vi "Calculate Joint Vectors.vi"(8 "Error In":errorcluster, 9 "Body Index":i32, 10 "Joints":T2, 11 "KinectSensor References":T3) -> (0 "Error Out":errorcluster, 1 "Joint 2-3 Vector":dbl[](array[numeric]), 2 "Joint 1-2 Vector":dbl[](array[numeric]), 3 "KinectSensor References":T3, 4 "Angle Between Bones (deg)":dbl)   [LabVIEW 2011, in "KinectOne.lvlib"]
doc: "Given 3 joints calculate the vector from joint 1 to 2 and from joint 2 to 3 as well as the angel between the two 'bone' vectors in degrees."
uses:
  KinectOne.lvlib
  Private/Type Defs/KinectSensor References.ctl
  Microsoft.Kinect
  C:/github/makerhub/KinectOne/LabVIEW/vi.lib/MakerHub/KinectOne/Private/Libs/BodyFrameDataInterface.dll
  Private/Libs/BodyFrameDataInterface.dll
  Private/Type Defs/JointType.ctl
  <vilib>/Analysis/baseanly.llb/Unit Vector (DBL).vi
  <vilib>/Analysis/NI_AALBase.lvlib
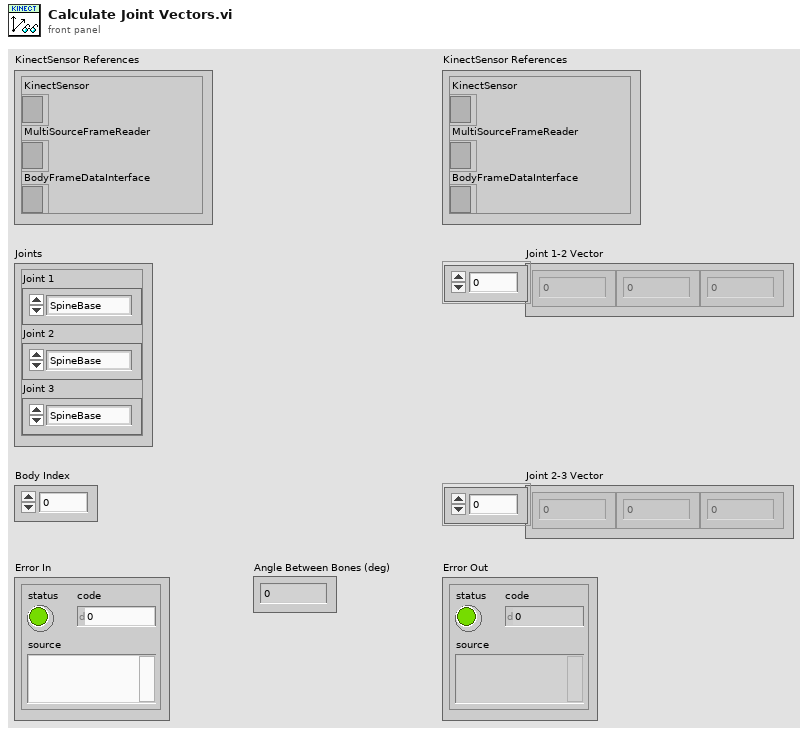
[diagram p1: front panel]
types:
  T1 = typedef "KinectOne.lvlib/JointType.ctl" = enum16{"SpineBase", "SpineMid", "Neck", "Head", "ShoulderLeft", "ElbowLeft", "WristLeft", "HandLeft", "ShoulderRight", "ElbowRight", "WristRight", "HandRight", "HipLeft", "KneeLeft", "AnkleLeft", "FootLeft", "HipRight", "KneeRight", "AnkleRight", "FootRight", "SpineShoulder", "HandTipLeft", "ThumbLeft", "HandTipRight", "ThumbRight"}
  T2 = cluster{"Joint 1":T1, "Joint 2":T1, "Joint 3":T1}
  T3 = typedef "KinectOne.lvlib/KinectSensor References.ctl" = cluster{"KinectSensor":refnum<k24>, "MultiSourceFrameReader":refnum<k24>, "BodyFrameDataInterface":refnum<k24>}
  T4 = typedef "KinectOne.lvlib/Joint Position.ctl" = cluster{"Camera Space":cluster{"X":dbl, "Y":dbl, "Z":dbl}, "Color Space":cluster{"X":dbl, "Y":dbl}, "Depth Space":cluster{"X":dbl, "Y":dbl}, "Tracking State":enum16{"NotTracked", "Inferred", "Tracked"}}
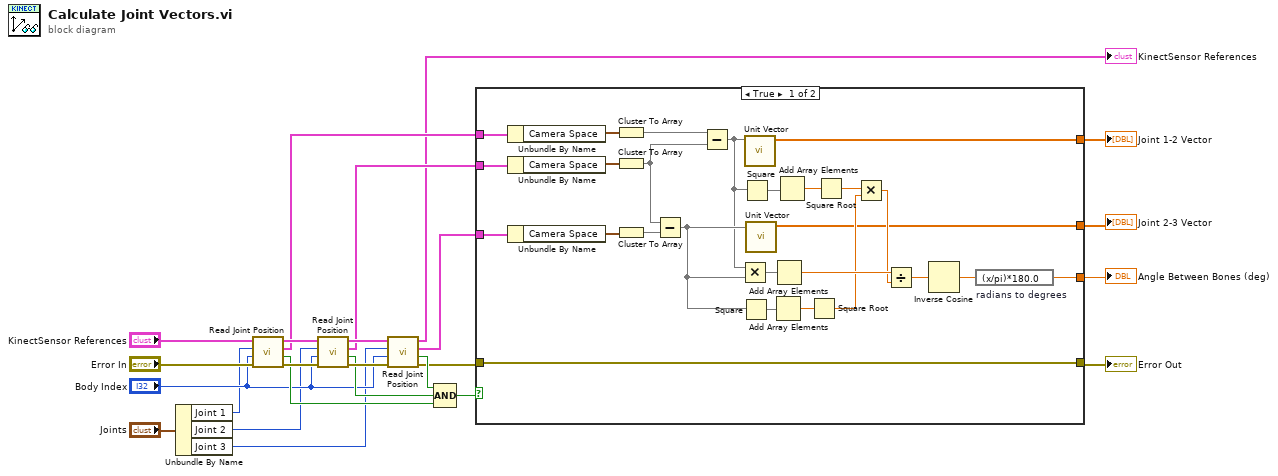
[diagram p0: block diagram]
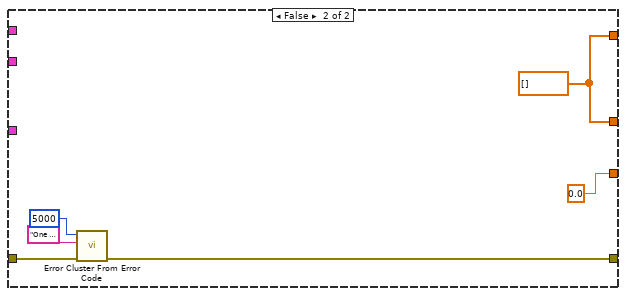
[diagram p2: hidden frame]
diagram:
  n1 = Unbundle By Name("Joints") -> ("Joint 1"=w3:T1, "Joint 2"=w2:T1, "Joint 3"=w1:T1)
  n2 = call "Read Joint Position.vi"("Error In"="Error In", "Body Index"="Body Index", "JointType"=w3, "KinectSensor References"="KinectSensor References") -> ("Error Out"=w22:errorcluster, "Tracked?"=w18:bool, "Joint Position"=w11:T4, "KinectSensor References"=w21:T3)  [unwired: 4 in]
  n3 = call "Read Joint Position.vi"("Error In"=w22, "Body Index"="Body Index", "JointType"=w2, "KinectSensor References"=w21) -> ("Error Out"=w20:errorcluster, "Tracked?"=w16:bool, "Joint Position"=w12:T4, "KinectSensor References"=w19:T3)  [unwired: 4 in]
  n4 = call "Read Joint Position.vi"("Error In"=w20, "Body Index"="Body Index", "JointType"=w1, "KinectSensor References"=w19) -> ("Error Out"=w14:errorcluster, "Tracked?"=w17:bool, "Joint Position"=w13:T4, "KinectSensor References"=→"KinectSensor References":T3)  [unwired: 4 in]
  n5 = Compound Arithmetic op=AND(w17, w16, w18) -> (w15:bool)
  n6 = case shown="True" w15 {
    tunnel: w14 -> [w25 w56]
    tunnel: w13 -> [w47 _]
    tunnel: w12 -> [w46 _]
    tunnel: w11 -> [w45 _]
    tunnel: [w29 w52] -> w8
    tunnel: [w28 w52] -> w7
    tunnel: [w26 0.0] -> w9
    tunnel: [w25 w53] -> w6
    frame True {
      n7 = Unbundle By Name(w45) -> ("Camera Space"=w48:cluster{"X":dbl, "Y":dbl, "Z":dbl})
      n8 = Unbundle By Name(w46) -> ("Camera Space"=w49:cluster{"X":dbl, "Y":dbl, "Z":dbl})
      n9 = Unbundle By Name(w47) -> ("Camera Space"=w50:cluster{"X":dbl, "Y":dbl, "Z":dbl})
      n10 = Cluster To Array(cluster=w48) -> (array=w32:dbl[])
      n11 = Cluster To Array(cluster=w49) -> (array=w31:dbl[])
      n12 = Cluster To Array(cluster=w50) -> (array=w30:dbl[])
      n13 = Subtract(x=w31, y=w30) -> (x-y=w44:dbl[])
      n14 = Subtract(x=w32, y=w31) -> (x-y=w43:dbl[])
      n15 = Multiply(x=w43, y=w44) -> (x*y=w41:dbl[])
      n16 = Square(x=w44) -> (x^2=w40:dbl[])
      n17 = Square(x=w43) -> (x^2=w39:dbl[])
      n18 = call-poly <vilib>:"Unit Vector.vi"("Input Vector"=w43) -> ("Unit Vector"=w29:dbl[])  [unwired: 8 in, 2 out]
      n19 = call-poly <vilib>:"Unit Vector.vi"("Input Vector"=w44) -> ("Unit Vector"=w28:dbl[])  [unwired: 8 in, 2 out]
      n20 = Add Array Elements(numeric array=w40) -> (sum=w34:dbl)
      n21 = Add Array Elements(numeric array=w41) -> (sum=w38:dbl)
      n22 = Add Array Elements(numeric array=w39) -> (sum=w33:dbl)
      n23 = Square Root(x=w34) -> (sqrt(x)=w35:dbl)
      n24 = Square Root(x=w33) -> (sqrt(x)=w42:dbl)
      n25 = Multiply(x=w42, y=w35) -> (x*y=w36:dbl)
      n26 = Divide(x=w38, y=w36) -> (x/y=w37:dbl)
      n27 = Inverse Cosine(1:w37) -> (0:w27:dbl)
      n28 = expression code="(x/pi)*180.0" "radians to degrees"(w27) -> (w26:dbl)
    }
    frame False {
      w52 = dbl[] [] ("Unit Vector")
      n29 = call <vilib>:"Error Cluster From Error Code.vi"("error in (no error)"=w56, "error message (\"\")"="One or more Joint not tracked, cannot calculate angle." ("error message (\"\")"), "error code (0)"=5000) -> ("error out"=w53:errorcluster)  [unwired: 6 in]
    }
  }
  "Error Out" <- w6
  "Angle Between Bones (deg)" <- w9
  "Joint 1-2 Vector" <- w8
  "Joint 2-3 Vector" <- w7
